vi "New Slide.vi"(6 "Offset":i32=1 min=1 step=1, 8 "error in (no error)":errorcluster, 9 "Type":T1=7 items=["Title Slide"=1, "Title and Content"=2, "Section Header"=3, "Two Content"=4, "Comparison"=5, "Title Only"=6, "Blank"=7], 10 "File refnum":refnum<k7>) -> (0 "error out":errorcluster, 1 "Slide refnum out":refnum<k7>, 2 "File refnum out":refnum<k7>)   [LabVIEW 2020, in "lvpptx.lvlib"]
uses:
  lvpptx.lvlib
  Slide Type.ctl
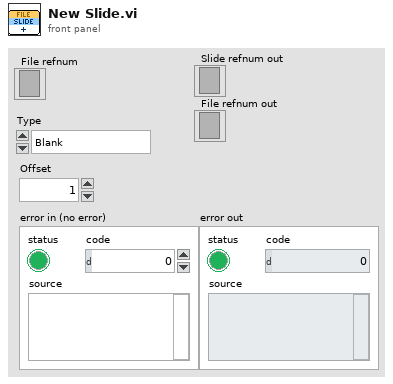
[diagram p1: front panel]
types:
  T1 = typedef "lvpptx.lvlib/Slide Type.ctl" = i32
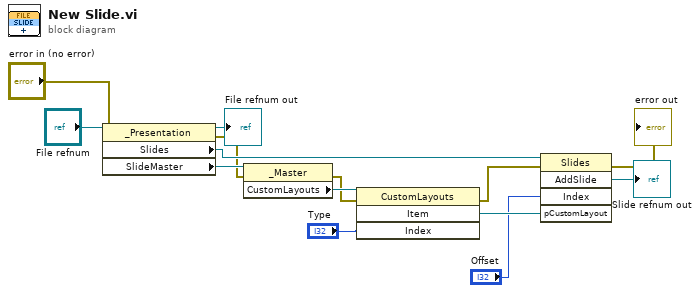
[diagram p0: block diagram]
diagram:
  n1 = property class="_Presentation"(reference="File refnum", error in="error in (no error)") -> (reference out=→"File refnum out":refnum<k7>, error out=w9:errorcluster, "Slides"=w10:refnum<k7>, "SlideMaster"=w13:refnum<k7>)
  n2 = property class="_Master"(reference=w13, error in=w9) -> (error out=w8:errorcluster, "CustomLayouts"=w12:refnum<k7>)  [unwired: 1 out]
  n3 = invoke class="CustomLayouts" method="Item"(reference=w12, error in=w8, "Index"="Type") -> (error out=w7:errorcluster, "Item"=w11:refnum<k7>)  [unwired: 1 in, 2 out]
  n4 = invoke class="Slides" method="AddSlide"(reference=w10, error in=w7, "Index"="Offset", "pCustomLayout"=w11) -> (error out=→"error out":errorcluster, "AddSlide"=→"Slide refnum out":refnum<k7>)  [unwired: 1 in, 3 out]
